vi "Banana_isNumericalType.vi"(10 "Allow Complex?":bool, 11 "type":T1) -> (3 "is Numeric":bool)   [LabVIEW 2021, in "Bananas.lvlib"]
uses:
  Bananas.lvlib
  <vilib>/Utility/Data Type/Type Definitions/Data Type.ctl
  <vilib>/Utility/Data Type/NI_Data Type.lvlib
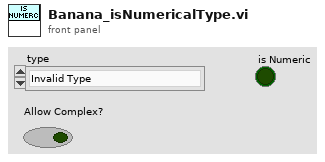
[diagram p1: front panel]
types:
  T1 = typedef "NI_Data Type.lvlib/Data Type.ctl" = enum8{"Invalid Type", "Void", "I8", "I16", "I32", "I64", "U8", "U16", "U32", "U64", "Single Float", "Double Float", "Extended Float", "Single Complex", "Double Complex", "Extended Complex", "Enum U8", "Enum U16", "Enum U32", "Enum U64", "Single Float With Unit", "Double Float With Unit", "Extended Float With Unit", "Single Complex with Unit", "Double Complex with Unit", "Extended Complex with Unit", "Boolean", "String", "Path", "Picture", "Tag", "Array", "Cluster", "Variant", "LV Variant", "Waveform", "Timestamp", "Digital Waveform", "Digital Data", "ExpressData", "Refnum", "External Data", "VI", "Poly VI", "LabVIEW Class Instance", "Fixed Point", "Set Collection", "Map Collection"}
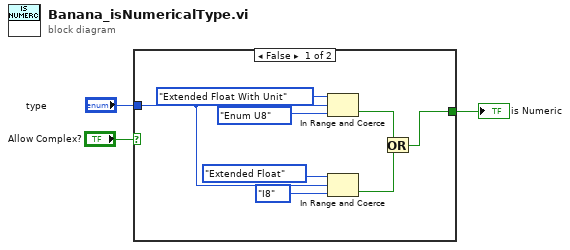
[diagram p0: block diagram]
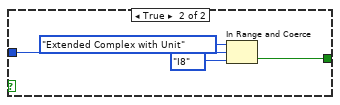
[diagram p2: hidden frame]
diagram:
  n1 = case shown="False" "Allow Complex?" {
    tunnel: "type" -> [w11 w15]
    tunnel: [w10 w14] -> w2
    frame False {
      n2 = In Range and Coerce(upper limit=Data_Type."Extended Float With Unit" ("type"), x=w11, lower limit=Data_Type."Enum U8" ("type")) -> (In Range?=w8:bool)  [unwired: 1 out]
      n3 = In Range and Coerce(upper limit=Data_Type."Extended Float" ("type"), x=w11, lower limit=Data_Type."I8" ("type")) -> (In Range?=w9:bool)  [unwired: 1 out]
      n4 = Or(x=w8, y=w9) -> (x .or. y?=w10:bool)
    }
    frame True {
      n5 = In Range and Coerce(upper limit=Data_Type."Extended Complex with Unit" ("type"), x=w15, lower limit=Data_Type."I8" ("type")) -> (In Range?=w14:bool)  [unwired: 1 out]
    }
  }
  "is Numeric" <- w2
